vi "udpLoop2.vi"(8 "error in (no error)":errorcluster) -> (0 "error out":errorcluster)   [LabVIEW 2015]
uses:
  <vilib>/DAQmx/read.llb/DAQmx Read (Counter DBL 1Chan 1Samp).vi
  <vilib>/DAQmx/miscellaneous.llb/DAQmx Fill In Error Info.vi
  <vilib>/GoldZinc Software/auzn custom VIs/CustomVI.lvlib
panel:
  in  "file path (use dialog)":path
  in  "Save":bool
  out "encoder":dbl format="%0.2f"
  in  "stop":bool
  out "Connections Attempted":i32
  out "Remote Port":u16
  out "Remote Address":string
  in  "Local Interface":string="10.10.20.1"
  in  "Local Port":u16=50000
  out "IMUvalues":dbl[](array[numeric])
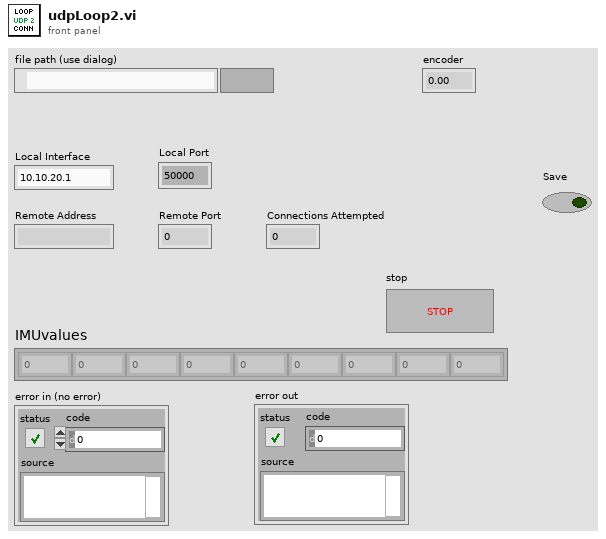
[diagram p1: front panel]
types:
  T1 = enum16{"open", "replace", "create", "open or create", "replace or create", "replace or create with confirmation"}
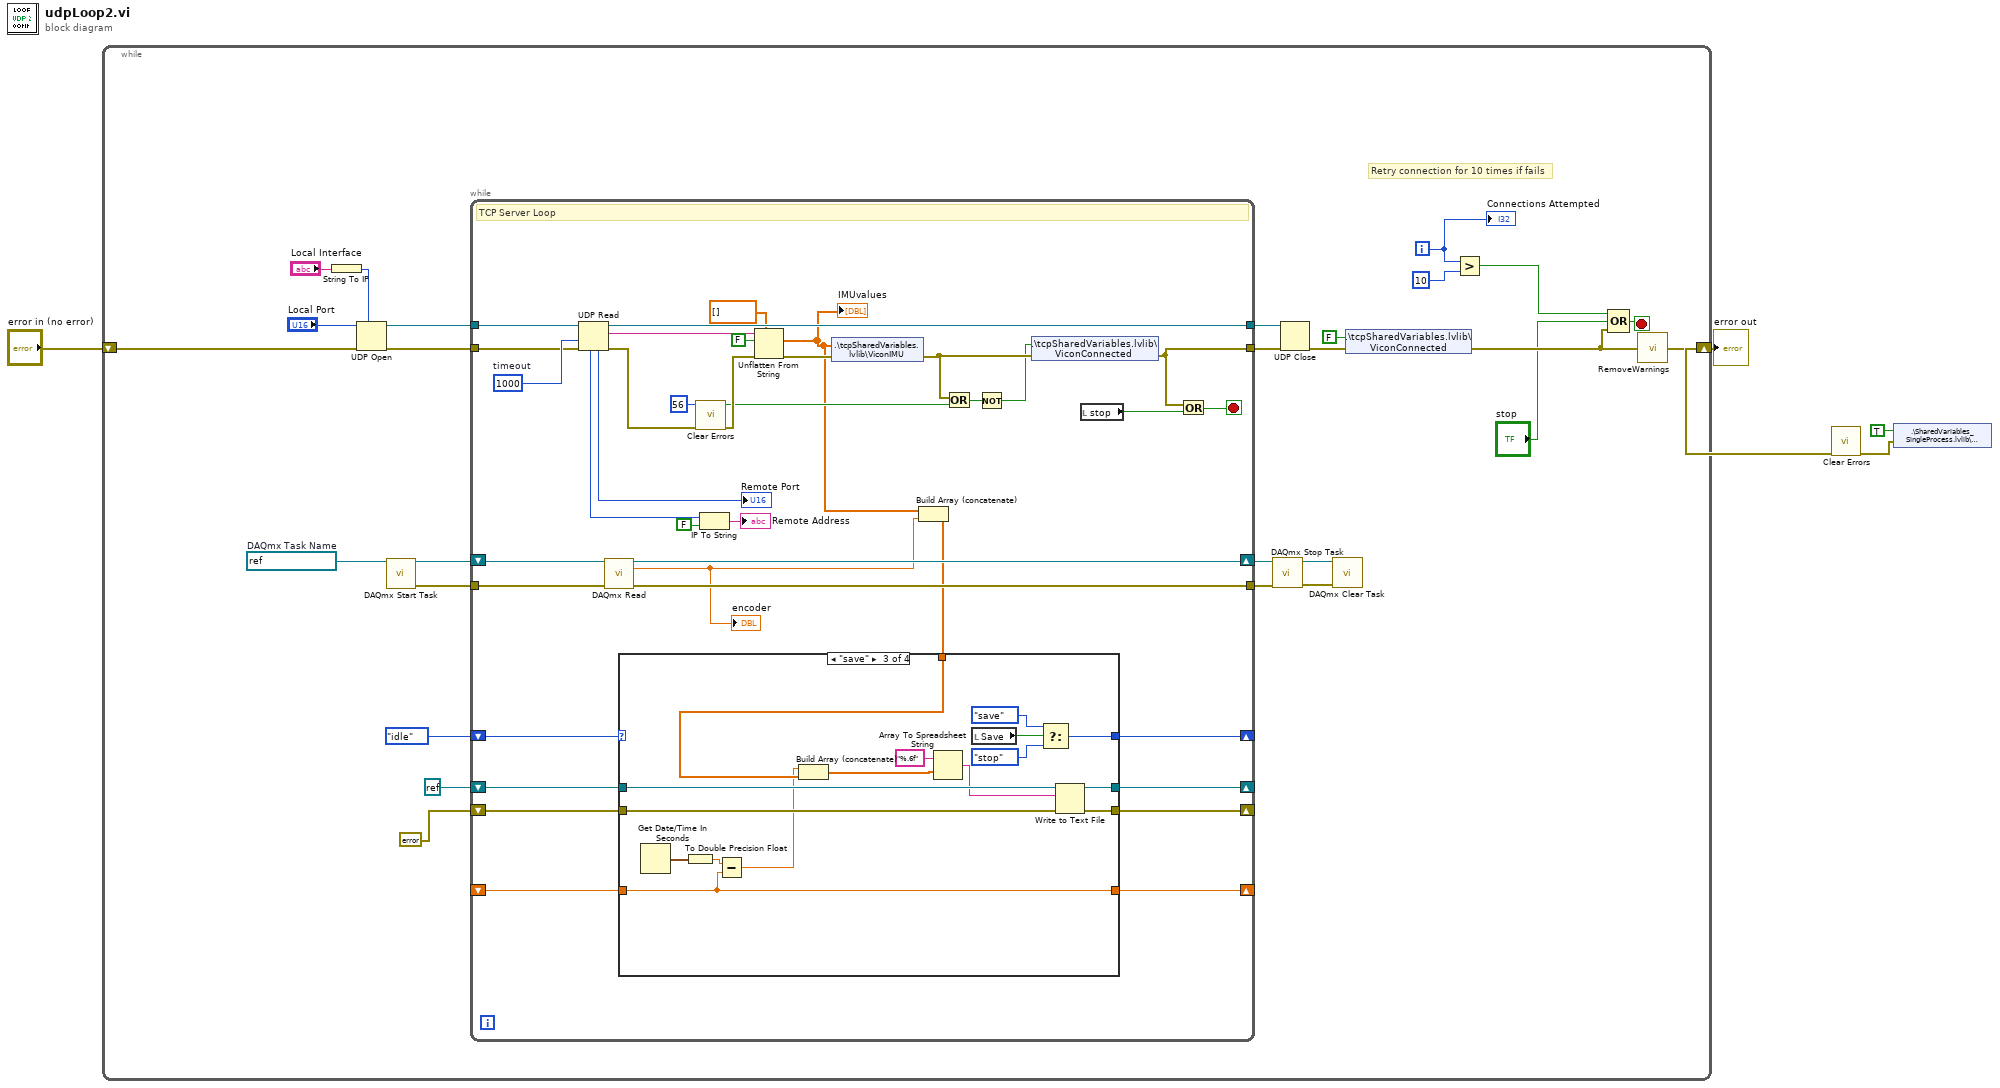
[diagram p0: block diagram]
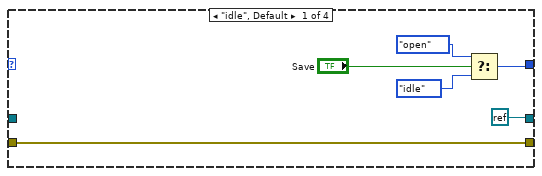
[diagram p2: hidden frame]
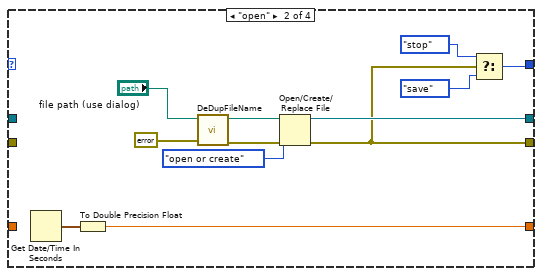
[diagram p3: hidden frame]
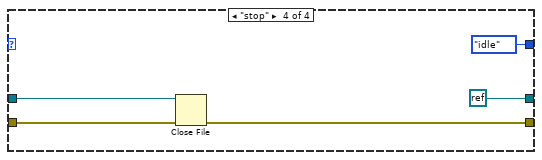
[diagram p4: hidden frame]
diagram:
  n1 = while {
    shift-right: [w17] -> w1
    shift-left: "error in (no error)" -> [w26]
    i -> [w20]
    stop <- w25 stop-if-true
    w14 = refnum<k21> "ctr0-PXI6363"  # DAQmx Task Name
    # "Retry connection for 10 times if fails"
    n2 = String To IP(1:"Local Interface") -> (0:w30:u32)
    n3 = UDP Open(7:w30, 8:w26, 11:"Local Port") -> (port=w23:refnum<k16>, 0:w22:errorcluster)  [unwired: 2 in, 1 out]
    n4 = call <vilib>:"DAQmx Start Task.vi"("task/channels in"=w14) -> ("task out"=w13:refnum<k21>, "error out"=w12:errorcluster)  [unwired: 13 in]
    n5 = while {
      tunnel: [w47] -> w31
      tunnel: [w68] -> w21
      tunnel: w23 -> [w66]
      tunnel: w22 -> [w65]
      tunnel: w12 -> [w45]
      shift-right: [w44] -> w11
      shift-left: w13 -> [w46]
      tunnel: [w43] -> w10
      shift-right: [w39] -> _
      shift-left: enum16{"idle", "open", "save", "stop"}."idle" -> [w40]
      shift-right: [w37] -> _
      shift-left: refnum<k0> refnum -> [w38]
      shift-right: [w35] -> _
      shift-left: errorcluster {"status"=FALSE, "code"=0, "source"=""} ("error out") -> [w36]
      shift-right: [w33] -> _
      shift-left: _ -> [w32]
      stop <- w53 stop-if-true
      w67 = 1000  # timeout
      # "TCP Server Loop"
      n6 = UDP Read(connection ID=w66, timeout ms (25000)=w67, 8:w65) -> (data out=w64:string, error out=w56:errorcluster, 3:w68:refnum<k16>, 4:→"Remote Port":u16, 6:w61:u32)  [unwired: 1 in]
      n7 = call-poly <vilib>:"DAQmx Read.vi"("task/channels in"=w46, "error in"=w45) -> ("task out"=w44:refnum<k21>, "data"=w41:dbl, "error out"=w43:errorcluster)  [unwired: 11 in]
      "encoder" <- w41
      n8 = call <vilib>:"Clear Errors.vi"("error in (no error)"=w56, "specific error code to clear (0: all)"=56) -> ("error out"=w54:errorcluster, "specific error cleared?"=w52:bool)  [unwired: 4 in]
      n9 = IP To String(1:FALSE ("dot notation? (F)"), 2:w61) -> (0:→"Remote Address":string)
      n10 = Unflatten From String(type=dbl[] [] ("Waveform Graph 2"), binary string=w64, data includes array or string size? (T)=FALSE, error in (no error)=w54) -> (value=w42:dbl[], error out=w57:errorcluster)  [unwired: 1 in, 1 out]
      "IMUvalues" <- w42
      n11 = shared-variable ".\\tcpSharedVariables.lvlib\\ViconIMU"(w42, error in=w57) -> (error out=w51:errorcluster)
      n12 = Build Array (concatenate)(w42, w41) -> (w34:dbl[])
      n13 = case shown="\"save\"" w40 {
        tunnel: [w73 w80 w100 enum16{"idle", "open", "save", "stop"}."idle"] -> w39
        tunnel: w38 -> [_ _ w95 w106]
        tunnel: [refnum<k0> refnum w86 w96 refnum<k0> refnum] -> w37
        tunnel: w36 -> [w69 _ w98 w105]
        tunnel: [w69 w78 w97 w104] -> w35
        tunnel: w34 -> [_ _ w91 _]
        tunnel: [_ w75 w87 _] -> w33
        tunnel: w32 -> [_ _ w87 _]
        frame "idle", Default {
          n14 = Select(t=enum16{"idle", "open", "save", "stop"}."open", s="Save", f=enum16{"idle", "open", "save", "stop"}."idle") -> (s? t:f=w73:enum16{"idle", "open", "save", "stop"})
        }
        frame "open" {
          n15 = Get Date/Time In Seconds() -> (seconds since 1Jan1904=w76:timestamp)
          n16 = To Double Precision Float(number=w76) -> (double precision float=w75:dbl)
          n17 = call <vilib>:"DeDupFileName.vi"("error in (no error)"=errorcluster {"status"=FALSE, "code"=0, "source"=""} ("error out"), "Path"="file path (use dialog)") -> ("error out"=w83:errorcluster, "Out Path"=w84:path)  [unwired: 7 in, 1 out]
          n18 = Open/Create/Replace File(file path (use dialog)=w84, error in=w83, operation (0:open)=T1."open or create") -> (refnum out=w86:refnum<file>, error out=w78:errorcluster)  [unwired: 3 in, 1 out]
          n19 = Select(t=enum16{"idle", "open", "save", "stop"}."stop", s=w78, f=enum16{"idle", "open", "save", "stop"}."save") -> (s? t:f=w80:enum16{"idle", "open", "save", "stop"})
        }
        frame "save" {
          n20 = Get Date/Time In Seconds() -> (seconds since 1Jan1904=w92:timestamp)
          n21 = To Double Precision Float(number=w92) -> (double precision float=w89:dbl)
          n22 = Subtract(x=w89, y=w87) -> (x-y=w88:dbl)
          n23 = Build Array (concatenate)(w88, w91) -> (w90:dbl[])
          n24 = Array To Spreadsheet String(array=w90, 3:"%.6f" ("format string")) -> (spreadsheet string=w94:string)  [unwired: 1 in]
          n25 = local read "Save"() -> (w99:bool)
          n26 = Select(t=enum16{"idle", "open", "save", "stop"}."save", s=w99, f=enum16{"idle", "open", "save", "stop"}."stop") -> (s? t:f=w100:enum16{"idle", "open", "save", "stop"})
          n27 = Write to Text File(file (use dialog)=w95, text=w94, error in=w98) -> (refnum out=w96:refnum<file>, error out=w97:errorcluster)  [unwired: 1 in, 1 out]
        }
        frame "stop" {
          n28 = Close File(refnum=w106, error in=w105) -> (error out=w104:errorcluster)  [unwired: 1 out]
        }
      }
      n29 = Or(x=w51, y=w52) -> (x .or. y?=w50:bool)
      n30 = Not(x=w50) -> (.not. x?=w49:bool)
      n31 = shared-variable ".\\tcpSharedVariables.lvlib\\ViconConnected"(w49, error in=w51) -> (error out=w47:errorcluster)
      n32 = local read "stop"() -> (w48:bool)
      n33 = Or(x=w47, y=w48) -> (x .or. y?=w53:bool)
    }
    n34 = call <vilib>:"DAQmx Stop Task.vi"("task/channels in"=w11, "error in"=w10) -> ("task out"=w9:refnum<k21>, "error out"=w8:errorcluster)  [unwired: 12 in]
    n35 = UDP Close(connection ID=w21, 8:w31) -> (error out=w28:errorcluster)  [unwired: 1 out]
    n36 = call <vilib>:"DAQmx Clear Task.vi"("task in"=w9, "error in"=w8) -> ()  [unwired: 13 in, 1 out]
    n37 = shared-variable ".\\tcpSharedVariables.lvlib\\ViconConnected"(FALSE ("Connected"), error in=w28) -> (error out=w16:errorcluster)
    n38 = Greater?(x=w20, y=10) -> (0:w18:bool)
    n39 = Compound Arithmetic op=OR(w18, "stop", w16) -> (w25:bool)
    n40 = call <vilib>:"RemoveWarnings.vi"("error in (no error)"=w16) -> ("error out"=w17:errorcluster)
    "Connections Attempted" <- w20
  }
  "error out" <- w1
  n41 = call <vilib>:"Clear Errors.vi"("error in (no error)"=w1) -> ("error out"=w2:errorcluster)  [unwired: 5 in, 1 out]
  n42 = shared-variable ".\\SharedVariables_SingleProcess.lvlib\\GlobalStop"(TRUE ("GlobalStop"), error in=w2) -> ()  [unwired: 1 out]
